vi "AliasTest.vi"(11 "MaxIndex":i32) -> (3 "Alias warning":bool)   [LabVIEW 2018]
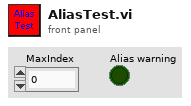
[diagram p1: front panel]
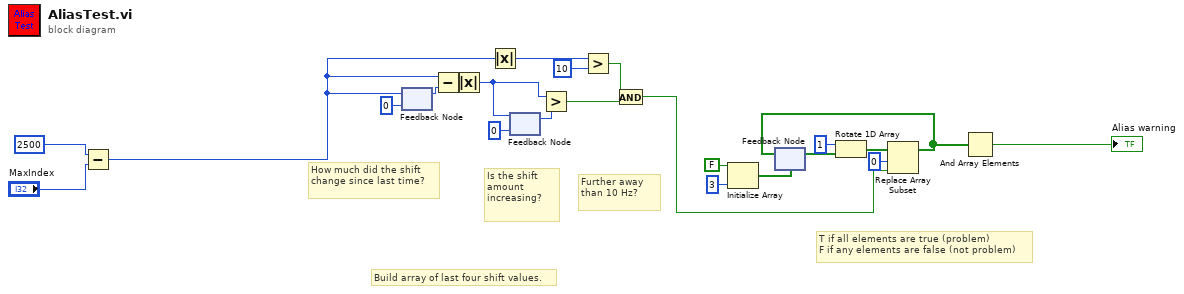
[diagram p0: block diagram]
diagram:
  # "T if all elements are true (problem)\nF if any elements are false (not problem)"
  # "Further away than 10 Hz?"
  # "Is the shift amount increasing?"
  # "How much did the shift change since last time?"
  # "Build array of last four shift values."
  n1 = Subtract(x=2500, y="MaxIndex") -> (x-y=w2:i32)
  n2 = feedback #1(0) -> (w10:i32)
  n3 = feedback-in #1(w2) -> ()
  n4 = Subtract(x=w2, y=w10) -> (x-y=w11:i32)
  n5 = Absolute Value(x=w11) -> (abs(x)=w18:i32)
  n6 = Absolute Value(x=w2) -> (abs(x)=w1:i32)
  n7 = feedback #2(0) -> (w12:i32)
  n8 = feedback-in #2(w18) -> ()
  n9 = Greater?(x=w18, y=w12) -> (0:w15:bool)
  n10 = Greater?(x=w1, y=10 ("x")) -> (0:w17:bool)
  n11 = And(x=w17, y=w15) -> (x .and. y?=w16:bool)
  n12 = Initialize Array(FALSE, 3 ("dimension size")) -> (w4:bool[])
  n13 = feedback #3(w4) -> (w5:bool[])
  n14 = Rotate 1D Array(1:w5, 2:1 ("n")) -> (0:w6:bool[])
  n15 = Replace Array Subset(array=w6, new element=w16, index=0) -> (w20:bool[])
  n16 = feedback-in #3(w20) -> ()
  n17 = And Array Elements(Boolean array=w20) -> (logical AND=→"Alias warning":bool)
